vi "Get Peripheral Info.vi"(8 "error in (no error)":errorcluster, 11 "FPGA Personality File Path":path) -> (0 "error out":errorcluster, 1 "Dimension of Channels":i32[](array[numeric]), 2 "Supported Peripherals":string[](array[string]), 3 "Duplicated FPGA Personality File Path":path)   [LabVIEW 2021, in "Personality.lvlib"]
doc: "Gets the peripheral information, such as supported peripherals and the number of the channels from the specified FPGA personality file."
uses:
  <vilib>/myRIO/Common/FPGA Personality Framework/Personality.lvlib
  <vilib>/xml/Load XML File.vi
  <vilib>/xml/Close Reference(Node).vi
  <vilib>/xml/NI_XML.lvlib
  <resource>/objmgr/DOMUserDefRef.rc
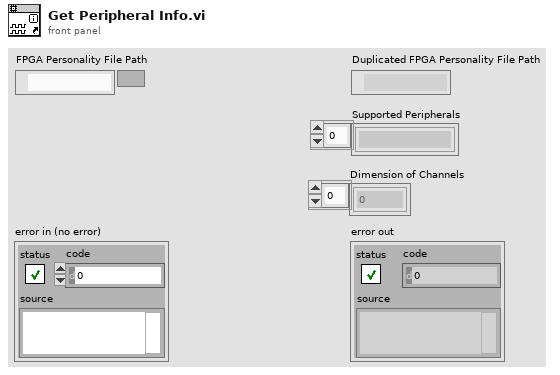
[diagram p1: front panel]
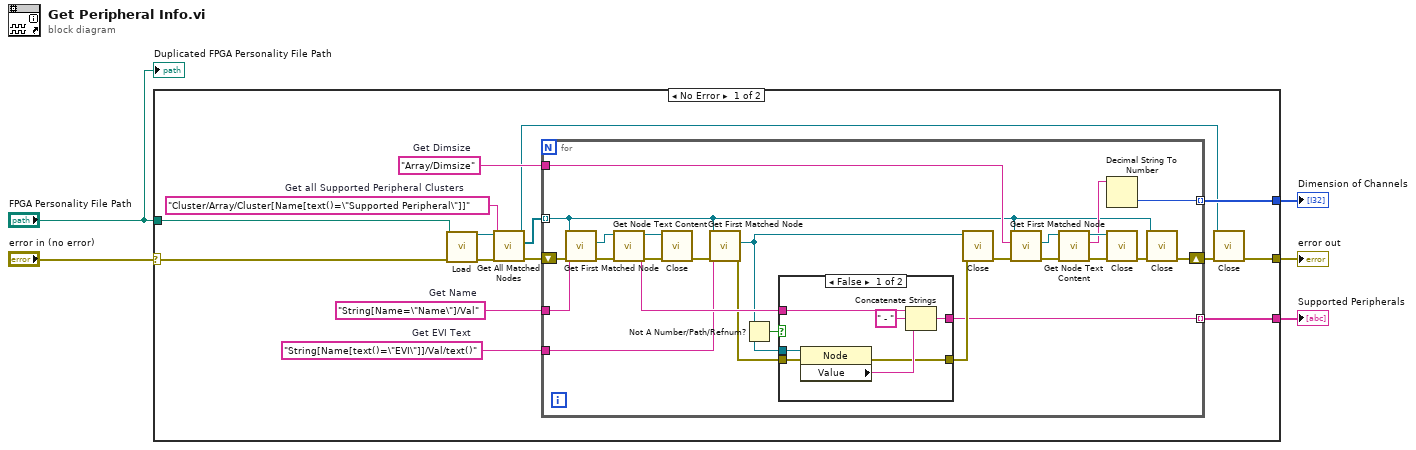
[diagram p0: block diagram]
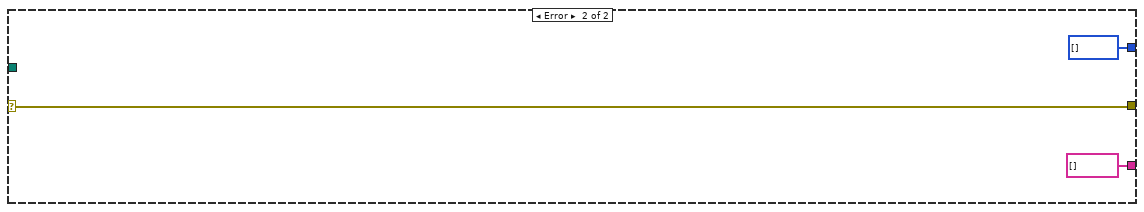
[diagram p3: hidden frame]
diagram:
  n1 = case shown="No Error" "error in (no error)" {
    selector: "error in (no error)" -> [w20 w57]
    tunnel: "FPGA Personality File Path" -> [w19 _]
    tunnel: [w10 i32[] []] -> w3
    tunnel: [w8 string[] []] -> w2
    tunnel: [w7 w57] -> w1
    frame No Error {
      w11 = "Array/Dimsize"  # Get Dimsize
      w13 = "String[Name=\"Name\"]/Val"  # Get Name
      w12 = "String[Name[text()=\"EVI\"]]/Val/text()"  # Get EVI Text
      w16 = "Cluster/Array/Cluster[Name[text()=\"Supported Peripheral\"]]"  # Get all Supported Peripheral Clusters
      n2 = call-poly <vilib>:"Load.vi"("path to XML document"=w19, "error in (no error)"=w20) -> ("DOM document out"=w18:refnum<k20>, "error out"=w17:errorcluster)  [unwired: 11 in, 1 out]
      n3 = call <vilib>:"Get All Matched Nodes.vi"("error in (no error)"=w17, "XPath expression"=w16, "node in"=w18) -> ("error out"=w14:errorcluster, "node result array"=w15:refnum<k20>[], "node out"=w6:refnum<k20>)  [unwired: 6 in]
      n4 = for {
        tunnel: w15 -> [w21] mode=indexing
        shift-right: [w22] -> w9
        shift-left: w14 -> [w45]
        tunnel: w13 -> [w44]
        tunnel: w12 -> [w37]
        tunnel: [w27] -> w8 mode=indexing
        tunnel: w11 -> [w26]
        tunnel: [w24] -> w10 mode=indexing
        n5 = call <vilib>:"Get First Matched Node.vi"("error in (no error)"=w45, "XPath expression"=w44, "node in"=w21) -> ("error out"=w42:errorcluster, "node result"=w43:refnum<k20>)  [unwired: 6 in, 1 out]
        n6 = call <vilib>:"Get Node Text Content.vi"("error in (no error)"=w42, "node in"=w43) -> ("error out"=w40:errorcluster, "node text"=w39:string, "node out"=w41:refnum<k20>)  [unwired: 7 in]
        n7 = call-poly <vilib>:"Close.vi"("error in (no error)"=w40, "node"=w41) -> ("error out"=w38:errorcluster)  [unwired: 7 in]
        n8 = call <vilib>:"Get First Matched Node.vi"("error in (no error)"=w38, "XPath expression"=w37, "node in"=w21) -> ("error out"=w35:errorcluster, "node result"=w33:refnum<k20>)  [unwired: 6 in, 1 out]
        n9 = Not A Number/Path/Refnum?(number/path/refnum=w33) -> (NaN/Path/Refnum?=w36:bool)
        n10 = case shown="False" w36 {
          tunnel: w39 -> [w52 w53]
          tunnel: w33 -> [w51 _]
          tunnel: [w48 w53] -> w27
          tunnel: w35 -> [w47 w54]
          tunnel: [w46 w54] -> w32
          frame False {
            n11 = property class="Node"(reference=w51, error in=w47) -> (error out=w46:errorcluster, "Value"=w49:string)  [unwired: 1 out]
            n12 = Concatenate Strings(w52, " - " ("string"), w49) -> (w48:string)
          }
          frame True {
          }
        }
        n13 = call-poly <vilib>:"Close.vi"("error in (no error)"=w32, "node"=w33) -> ("error out"=w34:errorcluster)  [unwired: 7 in]
        n14 = call <vilib>:"Get First Matched Node.vi"("error in (no error)"=w34, "XPath expression"=w26, "node in"=w21) -> ("error out"=w31:errorcluster, "node result"=w23:refnum<k20>)  [unwired: 6 in, 1 out]
        n15 = call <vilib>:"Get Node Text Content.vi"("error in (no error)"=w31, "node in"=w23) -> ("error out"=w29:errorcluster, "node text"=w25:string, "node out"=w30:refnum<k20>)  [unwired: 7 in]
        n16 = Decimal String To Number(string=w25) -> (number=w24:i32)  [unwired: 2 in, 1 out]
        n17 = call-poly <vilib>:"Close.vi"("error in (no error)"=w29, "node"=w30) -> ("error out"=w28:errorcluster)  [unwired: 7 in]
        n18 = call-poly <vilib>:"Close.vi"("error in (no error)"=w28, "node"=w21) -> ("error out"=w22:errorcluster)  [unwired: 7 in]
      }
      n19 = call-poly <vilib>:"Close.vi"("error in (no error)"=w9, "node"=w6) -> ("error out"=w7:errorcluster)  [unwired: 7 in]
    }
    frame Error {
    }
  }
  "Supported Peripherals" <- w2
  "Dimension of Channels" <- w3
  "error out" <- w1
  "Duplicated FPGA Personality File Path" <- "FPGA Personality File Path"
